vi "6_2.vi"() -> ()   [LabVIEW 2021, in "2023.lvlib"]
uses:
  2023.lvlib
panel:
  out "Result":i32
  in  "Demo / Real Input":bool
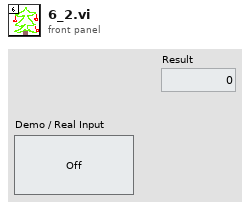
[diagram p1: front panel]
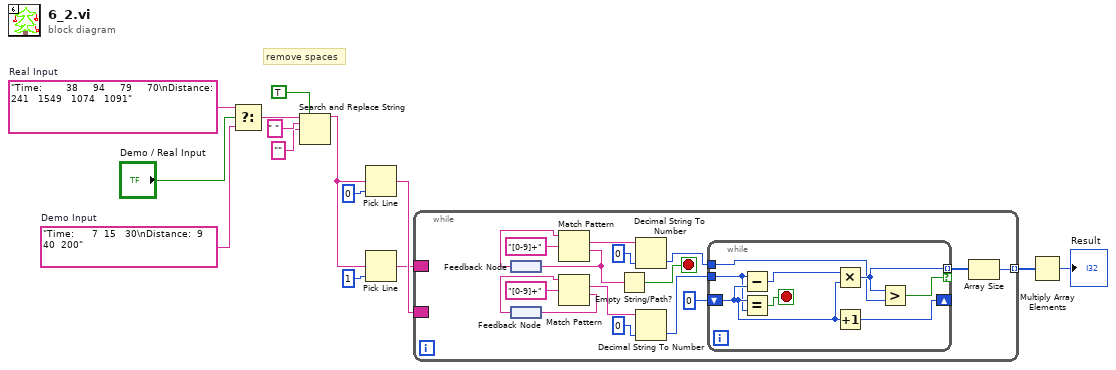
[diagram p0: block diagram]
diagram:
  w14 = "Time:        38     94     79     70\nDistance:   241   1549   1074   1091"  # Real Input
  w6 = "Time:      7  15   30\nDistance:  9  40  200"  # Demo Input
  # "remove spaces"
  n1 = Select(t=w14, s="Demo / Real Input", f=w6) -> (s? t:f=w2:string)
  n2 = Search and Replace String(replace all?=TRUE ("replace all? (F)"), input string=w2, search string=" ", replace string="" ("replace string (\"\")")) -> (result string=w1:string)  [unwired: 4 in, 3 out]
  n3 = Pick Line(multi-line string=w1, line index=0) -> (output string=w10:string)  [unwired: 1 in]
  n4 = Pick Line(multi-line string=w1, line index=1) -> (output string=w9:string)  [unwired: 1 in]
  n5 = while {
    border: w10 -> [_]
    border: w9 -> [_]
    tunnel: [w19] -> w8 mode=indexing
    stop <- w30 stop-if-true
    n6 = feedback #1() -> (w27:string)
    n7 = feedback #2() -> (w29:string)
    n8 = Match Pattern(string=w27, regular expression="[0-9]+" ("format string")) -> (match substring=w22:string, after substring=w25:string)  [unwired: 1 in, 2 out]
    n9 = feedback-in #1(w25) -> ()
    n10 = Match Pattern(string=w29, regular expression="[0-9]+" ("format string")) -> (match substring=w24:string, after substring=w23:string)  [unwired: 1 in, 2 out]
    n11 = feedback-in #2(w23) -> ()
    n12 = Empty String/Path?(string/path=w25) -> (empty?=w30:bool)
    n13 = Decimal String To Number(string=w22, default (0L)=i64 0 ("line index")) -> (number=w21:i64)  [unwired: 1 in, 1 out]
    n14 = Decimal String To Number(string=w24, default (0L)=i64 0 ("line index")) -> (number=w16:i64)  [unwired: 1 in, 1 out]
    n15 = while {
      tunnel: [w37] -> w20 mode=indexing if=w35
      tunnel: w21 -> [w36]
      tunnel: w16 -> [w32]
      shift-right: [w34] -> _
      shift-left: i64 0 ("line index") -> [w33]
      stop <- w31 stop-if-true
      n16 = Subtract(x=w32, y=w33) -> (x-y=w38:i64)
      n17 = Equal?(x=w33, y=w32) -> (x = y?=w31:bool)
      n18 = Multiply(x=w38, y=w33) -> (x*y=w37:i64)
      n19 = Increment(x=w33) -> (x+1=w34:i64)
      n20 = Greater?(x=w37, y=w36) -> (0:w35:bool)
    }
    n21 = Array Size(array=w20) -> (size(s)=w19:i32)
  }
  n22 = Multiply Array Elements(1:w8) -> (0:→"Result":i32)
